vi "hardware_optpumptester.vi"(8 "error in":errorcluster, 10 "Pump?":bool) -> (0 "error out":errorcluster)   [LabVIEW 2012]
uses:
  <vilib>/DAQmx/write.llb/DAQmx Write (Digital Wfm 1Chan NSamp).vi
  <vilib>/Waveform/DWDTOps.llb/Digital Pattern Generator (Single Value).vi
  <vilib>/DAQmx/create/channels.llb/DAQmx Create Channel (DO-Digital Output).vi
  <vilib>/Waveform/DWDTOps.llb/DWDT Append Digital Samples.vi
  <vilib>/Waveform/DWDTOps.llb/DWDT Digital Size.vi
  <vilib>/DAQmx/configure/timing.llb/DAQmx Timing (Sample Clock).vi
  <vilib>/Waveform/DWDTOps.llb/DWDT Uncompress Digital.vi
  <vilib>/DAQmx/miscellaneous.llb/DAQmx Fill In Error Info.vi
  <resource>/objmgr/daqmx.rc
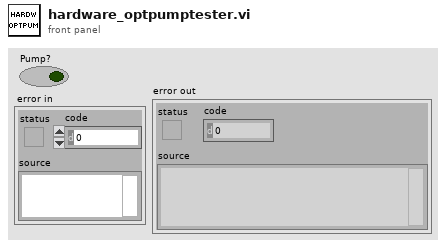
[diagram p1: front panel]
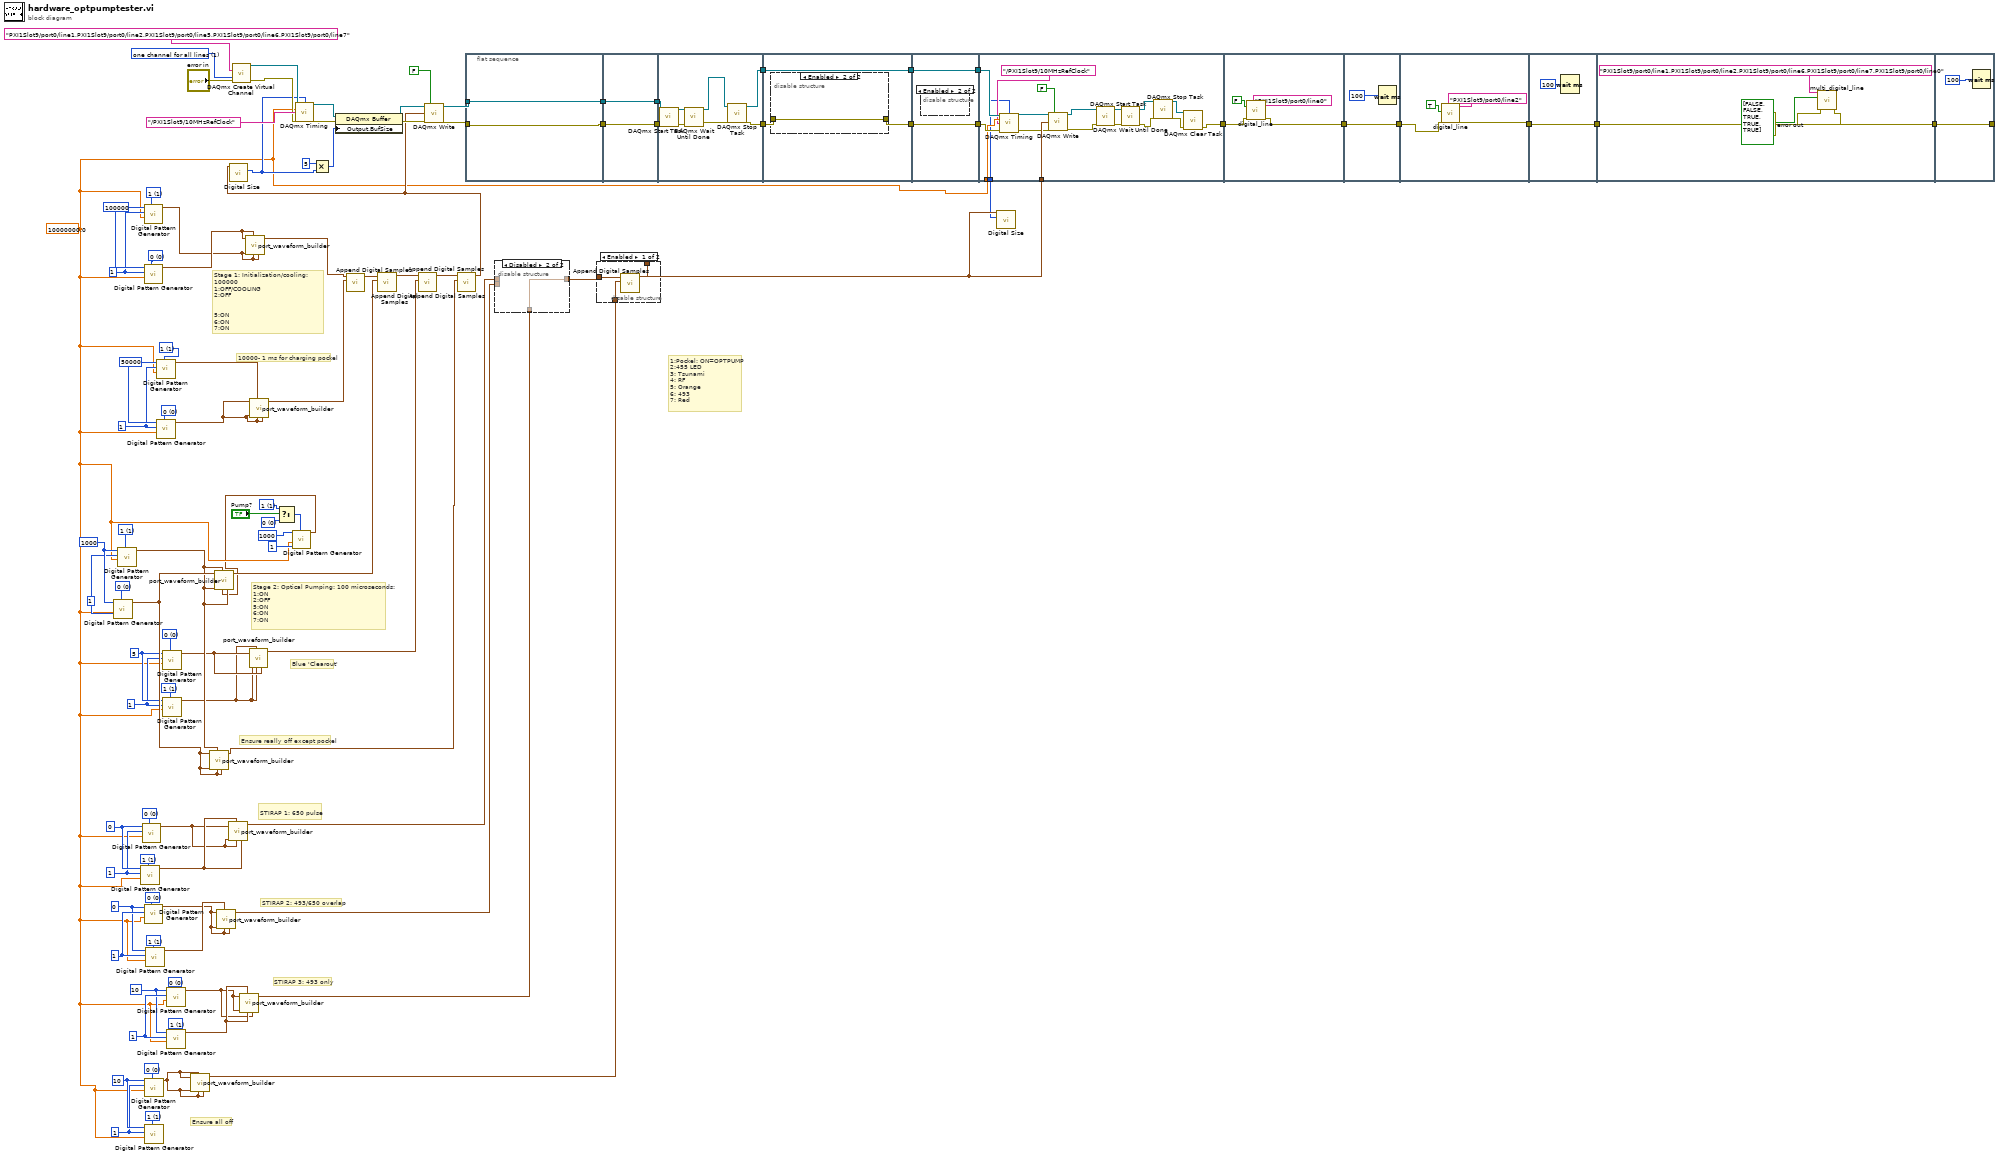
[diagram p0: block diagram]
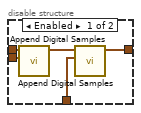
[diagram p2: hidden frame]
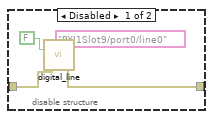
[diagram p4: hidden frame]
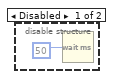
[diagram p5: hidden frame]
diagram:
  w20 = u32 10 ("number of samples")
  w23 = u8 1 items=["0", "1", "Z", "L", "H", "X", "T", "V"] ("value")
  w24 = u8 0 items=["0", "1", "Z", "L", "H", "X", "T", "V"] ("value")
  w25 = u32 1 ("number of signals")
  w26 = u32 0 ("number of samples")
  w27 = u8 1 items=["0", "1", "Z", "L", "H", "X", "T", "V"] ("value")
  w28 = u8 0 items=["0", "1", "Z", "L", "H", "X", "T", "V"] ("value")
  w29 = u32 1 ("number of signals")
  w50 = u8 0 items=["0", "1", "Z", "L", "H", "X", "T", "V"] ("value")
  w48 = u32 1 ("number of signals")
  w49 = u32 5 ("number of samples")
  w2 = u8 1 items=["0", "1", "Z", "L", "H", "X", "T", "V"] ("value")
  w62 = u8 0 items=["0", "1", "Z", "L", "H", "X", "T", "V"] ("value")
  w60 = u32 1 ("number of signals")
  w61 = u32 50000 ("number of samples")
  w63 = u8 1 items=["0", "1", "Z", "L", "H", "X", "T", "V"] ("value")
  w69 = u8 1 items=["0", "1", "Z", "L", "H", "X", "T", "V"] ("value")
  w68 = u8 0 items=["0", "1", "Z", "L", "H", "X", "T", "V"] ("value")
  w80 = u8 0 items=["0", "1", "Z", "L", "H", "X", "T", "V"] ("value")
  w78 = u32 1 ("number of signals")
  w79 = u32 10 ("number of samples")
  w81 = u8 1 items=["0", "1", "Z", "L", "H", "X", "T", "V"] ("value")
  w84 = u8 0 items=["0", "1", "Z", "L", "H", "X", "T", "V"] ("value")
  w82 = u32 1 ("number of signals")
  w83 = u32 0 ("number of samples")
  w1 = u8 1 items=["0", "1", "Z", "L", "H", "X", "T", "V"] ("value")
  w89 = u8 0 items=["0", "1", "Z", "L", "H", "X", "T", "V"] ("value")
  w85 = u32 1 ("number of signals")
  w86 = u32 1000 ("number of samples")
  w90 = u8 1 items=["0", "1", "Z", "L", "H", "X", "T", "V"] ("value")
  w91 = u8 0 items=["0", "1", "Z", "L", "H", "X", "T", "V"] ("value")
  w87 = u32 1 ("number of signals")
  w88 = u32 100000 ("number of samples")
  w92 = u8 1 items=["0", "1", "Z", "L", "H", "X", "T", "V"] ("value")
  w97 = 1 items=["one channel for each line", "one channel for all lines"] ("line grouping")
  w19 = 10000000.0 ("rate")
  # "Blue 'Clearout'"
  # "10000- 1 ms for charging pockel"
  # "STIRAP 3: 493 only"
  # "STIRAP 2: 493/650 overlap"
  # "Ensure really off except pockel"
  # "Ensure all off"
  # "STIRAP 1: 650 pulse"
  # "Stage 2: Optical Pumping: 100 microseconds: \n1:ON\n2:OFF\n5:ON\n6:ON\n7:ON"
  # "Stage 1: Initialization/cooling: 100000\n1:OFF/COOLING\n2:OFF\n\n\n5:ON\n6:ON\n7:ON"
  # "1:Pockel: ON=OPTPUMP\n2:455 LED\n3: Tsunami\n4: RF\n5: Orange\n6: 493\n7: Red"
  n1 = call-poly <vilib>:"Digital Pattern Generator.vi"("value"=w89, "sample rate"=w19, "number of signals"=w85, "number of samples"=w86) -> ("digital waveform"=w54:digitalwaveform)  [unwired: 6 in, 1 out]
  n2 = call-poly <vilib>:"Digital Pattern Generator.vi"("value"=w90, "sample rate"=w19, "number of signals"=w85, "number of samples"=w86) -> ("digital waveform"=w30:digitalwaveform)  [unwired: 6 in, 1 out]
  n3 = call-poly <vilib>:"Digital Pattern Generator.vi"("value"=w1, "sample rate"=w19, "number of signals"=w82, "number of samples"=w83) -> ("digital waveform"=w18:digitalwaveform)  [unwired: 6 in, 1 out]
  n4 = call-poly <vilib>:"Digital Pattern Generator.vi"("value"=w84, "sample rate"=w19, "number of signals"=w82, "number of samples"=w83) -> ("digital waveform"=w17:digitalwaveform)  [unwired: 6 in, 1 out]
  n5 = call-poly <vilib>:"Digital Pattern Generator.vi"("value"=w92, "sample rate"=w19, "number of signals"=w87, "number of samples"=w88) -> ("digital waveform"=w71:digitalwaveform)  [unwired: 6 in, 1 out]
  n6 = call-poly <vilib>:"Digital Pattern Generator.vi"("value"=w91, "sample rate"=w19, "number of signals"=w87, "number of samples"=w88) -> ("digital waveform"=w72:digitalwaveform)  [unwired: 6 in, 1 out]
  n7 = call-poly <vilib>:"Digital Pattern Generator.vi"("value"=w28, "sample rate"=w19, "number of signals"=w29, "number of samples"=w26) -> ("digital waveform"=w7:digitalwaveform)  [unwired: 6 in, 1 out]
  n8 = call-poly <vilib>:"Digital Pattern Generator.vi"("value"=w80, "sample rate"=w19, "number of signals"=w78, "number of samples"=w79) -> ("digital waveform"=w51:digitalwaveform)  [unwired: 6 in, 1 out]
  n9 = call-poly <vilib>:"Digital Pattern Generator.vi"("value"=w81, "sample rate"=w19, "number of signals"=w78, "number of samples"=w79) -> ()  [unwired: 6 in, 2 out]
  n10 = call-poly <vilib>:"Digital Pattern Generator.vi"("value"=w27, "sample rate"=w19, "number of signals"=w29, "number of samples"=w26) -> ("digital waveform"=w8:digitalwaveform)  [unwired: 6 in, 1 out]
  n11 = call-poly <vilib>:"Digital Pattern Generator.vi"("value"=w63, "sample rate"=w19, "number of signals"=w60, "number of samples"=w61) -> ("digital waveform"=w59:digitalwaveform)  [unwired: 6 in, 1 out]
  n12 = call-poly <vilib>:"Digital Pattern Generator.vi"("value"=w62, "sample rate"=w19, "number of signals"=w60, "number of samples"=w61) -> ("digital waveform"=w58:digitalwaveform)  [unwired: 6 in, 1 out]
  n13 = call-poly <vilib>:"Digital Pattern Generator.vi"("value"=w50, "sample rate"=w19, "number of signals"=w48, "number of samples"=w49) -> ("digital waveform"=w6:digitalwaveform)  [unwired: 6 in, 1 out]
  n14 = call-poly <vilib>:"Digital Pattern Generator.vi"("value"=w2, "sample rate"=w19, "number of signals"=w48, "number of samples"=w49) -> ("digital waveform"=w4:digitalwaveform)  [unwired: 6 in, 1 out]
  n15 = call-poly <vilib>:"Digital Pattern Generator.vi"("value"=w24, "sample rate"=w19, "number of signals"=w25, "number of samples"=w20) -> ("digital waveform"=w21:digitalwaveform)  [unwired: 6 in, 1 out]
  n16 = call-poly <vilib>:"Digital Pattern Generator.vi"("value"=w23, "sample rate"=w19, "number of signals"=w25, "number of samples"=w20) -> ("digital waveform"=w22:digitalwaveform)  [unwired: 6 in, 1 out]
  n17 = call "port_waveform_builder.vi"("Line 7"=w51, "Line 6"=w51, "Line 1"=w51, "Line 5"=w51, "Line 2"=w51) -> ("digital waveform out"=w76:digitalwaveform)  [unwired: 6 in]
  n18 = call "port_waveform_builder.vi"("Line 7"=w54, "Line 6"=w54, "Line 1"=w30, "Line 5"=w54, "Line 2"=w54) -> ("digital waveform out"=w14:digitalwaveform)  [unwired: 6 in]
  n19 = call "port_waveform_builder.vi"("Line 7"=w7, "Line 6"=w7, "Line 1"=w8, "Line 5"=w7, "Line 2"=w7) -> ("digital waveform out"=w15:digitalwaveform)  [unwired: 6 in]
  n20 = call "port_waveform_builder.vi"("Line 7"=w18, "Line 6"=w17, "Line 1"=w18, "Line 5"=w17, "Line 2"=w17) -> ("digital waveform out"=w16:digitalwaveform)  [unwired: 6 in]
  n21 = call-poly <vilib>:"DAQmx Create Virtual Channel.vi"("lines"=tag "PXI1Slot9/port0/line1,PXI1Slot9/port0/line2,PXI1Slot9/port0/line5,PXI1Slot9/port0/line6,PXI1Slot9/port0/line7", "line grouping"=w97, "error in"="error in") -> ("task out"=w98:refnum<k21>, "error out"=w95:errorcluster)  [unwired: 11 in]
  n22 = call "port_waveform_builder.vi"("Line 7"=w21, "Line 6"=w22, "Line 1"=w22, "Line 5"=w21, "Line 2"=w21) -> ("digital waveform out"=w12:digitalwaveform)  [unwired: 6 in]
  n23 = call "port_waveform_builder.vi"("Line 7"=w71, "Line 6"=w71, "Line 1"=w72, "Line 5"=w71, "Line 2"=w72) -> ("digital waveform out"=w57:digitalwaveform)  [unwired: 6 in]
  n24 = call "port_waveform_builder.vi"("Line 7"=w6, "Line 6"=w4, "Line 1"=w4, "Line 5"=w4, "Line 2"=w6) -> ("digital waveform out"=w46:digitalwaveform)  [unwired: 6 in]
  n25 = call "port_waveform_builder.vi"("Line 7"=w58, "Line 6"=w58, "Line 1"=w59, "Line 5"=w58, "Line 2"=w58) -> ("digital waveform out"=w56:digitalwaveform)  [unwired: 6 in]
  n26 = Select(t=w69, s="Pump?", f=w68) -> (s? t:f=w65:u8)
  n27 = call-poly <vilib>:"Digital Pattern Generator.vi"("value"=w65, "sample rate"=w19, "number of signals"=u32 1, "number of samples"=u32 1000) -> ("digital waveform"=w5:digitalwaveform)  [unwired: 6 in, 1 out]
  n28 = call "port_waveform_builder.vi"("Line 7"=w30, "Line 6"=w5, "Line 1"=w30, "Line 5"=w30, "Line 2"=w54) -> ("digital waveform out"=w77:digitalwaveform)  [unwired: 6 in]
  n29 = call-poly <vilib>:"Append Digital Samples.vi"("digital waveform B"=w56, "digital waveform A"=w57) -> ("digital waveform out"=w55:digitalwaveform)  [unwired: 8 in, 1 out]
  n30 = call-poly <vilib>:"Append Digital Samples.vi"("digital waveform B"=w77, "digital waveform A"=w55) -> ("digital waveform out"=w47:digitalwaveform)  [unwired: 8 in, 1 out]
  n31 = call-poly <vilib>:"Append Digital Samples.vi"("digital waveform B"=w46, "digital waveform A"=w47) -> ("digital waveform out"=w3:digitalwaveform)  [unwired: 8 in, 1 out]
  n32 = call-poly <vilib>:"Append Digital Samples.vi"("digital waveform B"=w14, "digital waveform A"=w3) -> ("digital waveform out"=w38:digitalwaveform)  [unwired: 8 in, 1 out]
  n33 = call-poly <vilib>:"Digital Size.vi"("digital waveform in"=w38) -> ("number of samples"=w33:i32)  [unwired: 7 in, 3 out]
  n34 = call-poly <vilib>:"DAQmx Timing.vi"("task/channels in"=w98, "samples per channel"=w33, "rate"=w19, "source"=tag "/PXI1Slot9/10MHzRefClock", "error in"=w95) -> ("task out"=w103:refnum<k21>, "error out"=w102:errorcluster)  [unwired: 9 in]
  n35 = Multiply(x=5, y=w33) -> (x*y=w40:i32)
  n36 = property class="DAQmx Buffer"(reference=w103, error in=w102, "Output.BufSize"=w40) -> (reference out=w100:refnum<k21>, error out=w94:errorcluster)
  n37 = call-poly <vilib>:"DAQmx Write.vi"("task/channels in"=w100, "auto start"=FALSE, "data"=w38, "error in"=w94) -> ("task out"=w99:refnum<k21>, "error out"=w93:errorcluster)  [unwired: 9 in, 1 out]
  n38 = flat-sequence {
    tunnel: w93 -> [w105]
    tunnel: w99 -> [w106]
    tunnel: [w106] -> w44
    tunnel: [w105] -> w41
    tunnel: w44 -> [w108]
    tunnel: [w108] -> w43
    tunnel: [w107] -> w42
    tunnel: w41 -> [w107]
    tunnel: w43 -> [w116]
    tunnel: w42 -> [w115]
    tunnel: [w112] -> w35
    tunnel: [w111] -> w34
    tunnel: [w119] -> w53
    tunnel: [w117] -> w36
    tunnel: w35 -> [w117]
    tunnel: w34 -> [w118]
    tunnel: w53 -> [w126]
    tunnel: [w126] -> w39
    tunnel: [w125] -> w37
    tunnel: w36 -> [w125]
    tunnel: w39 -> [w134]
    tunnel: [w135] -> w10
    tunnel: w37 -> [w131]
    tunnel: w32 -> [w145]
    tunnel: w19 -> [w130]
    tunnel: w31 -> [w128]
    tunnel: w10 -> [w146]
    tunnel: [w147] -> w9
    tunnel: w9 -> [w151]
    tunnel: [w151] -> w11
    tunnel: [w152] -> w52
    tunnel: w11 -> [w153]
    tunnel: w52 -> [w157]
    tunnel: [w157] -> w70
    tunnel: w70 -> [w161]
    tunnel: [w160] -> w45
    tunnel: [w163] -> w74
    tunnel: w45 -> [w163]
    frame #0 {
    }
    frame #1 {
    }
    frame #2 {
      n39 = call <vilib>:"DAQmx Start Task.vi"("task/channels in"=w116, "error in"=w115) -> ("task out"=w113:refnum<k21>, "error out"=w114:errorcluster)  [unwired: 12 in]
      n40 = call <vilib>:"DAQmx Wait Until Done.vi"("task/channels in"=w113, "error in"=w114) -> ("task out"=w109:refnum<k21>, "error out"=w110:errorcluster)  [unwired: 12 in]
      n41 = call <vilib>:"DAQmx Stop Task.vi"("task/channels in"=w109, "error in"=w110) -> ("task out"=w112:refnum<k21>, "error out"=w111:errorcluster)  [unwired: 12 in]
    }
    frame #3 {
      n42 = disable-structure shown="Enabled" {
        disable-tunnel: [w123 w124] -> w119
        disable-tunnel: w118 -> [w122 w124]
        frame Disabled {
          n43 = call "digital_line.vi"("error in"=w122, "Boolean"=FALSE, "lines"=tag "PXI1Slot9/port0/line0") -> ("error out"=w123:errorcluster)  [unwired: 4 in]
        }
        frame Enabled {
        }
      }
    }
    frame #4 {
      n44 = disable-structure shown="Enabled" {
        frame Disabled {
          n45 = Wait (ms)(milliseconds to wait=u32 50) -> ()  [unwired: 1 out]
        }
        frame Enabled {
        }
      }
    }
    frame #5 {
      n46 = call-poly <vilib>:"DAQmx Timing.vi"("task/channels in"=w131, "samples per channel"=w128, "rate"=w130, "source"=tag "/PXI1Slot9/10MHzRefClock", "error in"=w134) -> ("task out"=w132:refnum<k21>, "error out"=w133:errorcluster)  [unwired: 9 in]
      n47 = call-poly <vilib>:"DAQmx Write.vi"("task/channels in"=w132, "auto start"=FALSE, "data"=w145, "error in"=w133) -> ("task out"=w143:refnum<k21>, "error out"=w136:errorcluster)  [unwired: 9 in, 1 out]
      n48 = call <vilib>:"DAQmx Start Task.vi"("task/channels in"=w143, "error in"=w136) -> ("task out"=w142:refnum<k21>, "error out"=w137:errorcluster)  [unwired: 12 in]
      n49 = call <vilib>:"DAQmx Wait Until Done.vi"("task/channels in"=w142, "error in"=w137) -> ("task out"=w141:refnum<k21>, "error out"=w138:errorcluster)  [unwired: 12 in]
      n50 = call <vilib>:"DAQmx Stop Task.vi"("task/channels in"=w141, "error in"=w138) -> ("task out"=w140:refnum<k21>, "error out"=w139:errorcluster)  [unwired: 12 in]
      n51 = call <vilib>:"DAQmx Clear Task.vi"("task in"=w140, "error in"=w139) -> ("error out"=w135:errorcluster)  [unwired: 13 in]
    }
    frame #6 {
      n52 = call "digital_line.vi"("error in"=w146, "Boolean"=FALSE, "lines"=tag "PXI1Slot9/port0/line0") -> ("error out"=w147:errorcluster)  [unwired: 4 in]
    }
    frame #7 {
      n53 = Wait (ms)(milliseconds to wait=u32 100) -> ()  [unwired: 1 out]
    }
    frame #8 {
      n54 = call "digital_line.vi"("error in"=w153, "Boolean"=TRUE, "lines"=tag "PXI1Slot9/port0/line2") -> ("error out"=w152:errorcluster)  [unwired: 4 in]
    }
    frame #9 {
      n55 = Wait (ms)(milliseconds to wait=u32 100) -> ()  [unwired: 1 out]
    }
    frame #10 {
      n56 = call "multi_digital_line.vi"("error in"=w161, "data"=bool[] [FALSE, FALSE, TRUE, TRUE, TRUE], "lines"=tag "PXI1Slot9/port0/line1,PXI1Slot9/port0/line2,PXI1Slot9/port0/line6,PXI1Slot9/port0/line7,PXI1Slot9/port0/line0") -> ("error out"=w160:errorcluster)  [unwired: 8 in]
    }
    frame #11 {
      n57 = Wait (ms)(milliseconds to wait=u32 100) -> ()  [unwired: 1 out]
    }
  }
  n58 = disable-structure shown="Disabled" {
    disable-tunnel: w16 -> [w168 _]
    disable-tunnel: w15 -> [w167 _]
    disable-tunnel: [w165 w169] -> w13
    disable-tunnel: w12 -> [w164 w169]
    frame Enabled {
      n59 = call-poly <vilib>:"Append Digital Samples.vi"("digital waveform B"=w167, "digital waveform A"=w168) -> ("digital waveform out"=w166:digitalwaveform)  [unwired: 8 in, 1 out]
      n60 = call-poly <vilib>:"Append Digital Samples.vi"("digital waveform B"=w164, "digital waveform A"=w166) -> ("digital waveform out"=w165:digitalwaveform)  [unwired: 8 in, 1 out]
    }
    frame Disabled {
    }
  }
  n61 = disable-structure shown="Enabled" {
    disable-tunnel: w76 -> [w172 _]
    disable-tunnel: [w171 w173] -> w32
    disable-tunnel: w13 -> [w170 w173]
    frame Enabled {
      n62 = call-poly <vilib>:"Append Digital Samples.vi"("digital waveform B"=w172, "digital waveform A"=w170) -> ("digital waveform out"=w171:digitalwaveform)  [unwired: 8 in, 1 out]
    }
    frame Disabled {
    }
  }
  n63 = call-poly <vilib>:"Digital Size.vi"("digital waveform in"=w32) -> ("number of samples"=w31:i32)  [unwired: 7 in, 3 out]
  "error out" <- w74
